vi "Parse Core.vi"(0 "SG Path in":refnum<class "SG 18GHz Path.lvclass">, 5 "Config Row":string[](array[string]), 11 "error in":errorcluster) -> (4 "SG Path out":refnum<class "SG 18GHz Path.lvclass">, 15 "error out":errorcluster)   [LabVIEW 2023, in "RFFixtureCharact.RFPM.lvlib" / "SG 18GHz Path.lvclass"]
uses:
  SG 18GHz Path.lvclass
  C:/srd-semi-rfcal-software/AuxTools/STSRFFixtureCharactUtility/Source/Code Modules/Common/Base Classes/Path/Path.lvclass
  Charact Result Accessor/Scalar/Scalar Charact Result Accessor.lvclass
  C:/srd-semi-rfcal-software/AuxTools/STSRFFixtureCharactUtility/Source/Code Modules/Fixture/RFPM/Charact Result Accessor/Base/Charact Result Accessor.lvclass
  C:/srd-semi-rfcal-software/AuxTools/STSRFFixtureCharactUtility/Source/Code Modules/Common/Result Accessor/Result Accessor.lvclass
  Common/Base Classes/Path/Path.lvclass/Path.ctl
  Common/Base Classes/Path/Properties/Read Date.vi
  Common/Base Classes/Path/Properties/Read Interval.vi
  Common/Data Cache/Settings Dictionary/Setting Keys.vi
  Public/Base Classes/Scalar/SG Abstract Path/SG Abstract Path.lvclass
  Common/RFCalAndFixtureCharact.Common.lvlib
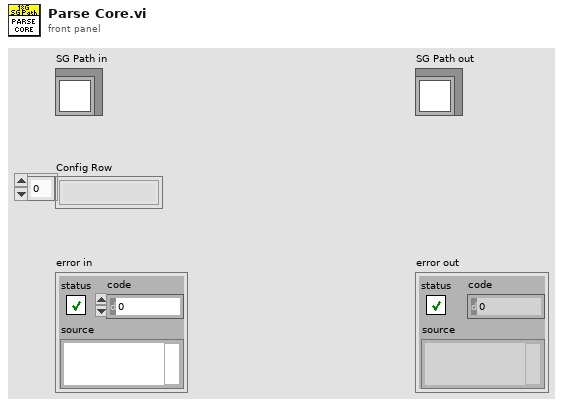
[diagram p1: front panel]
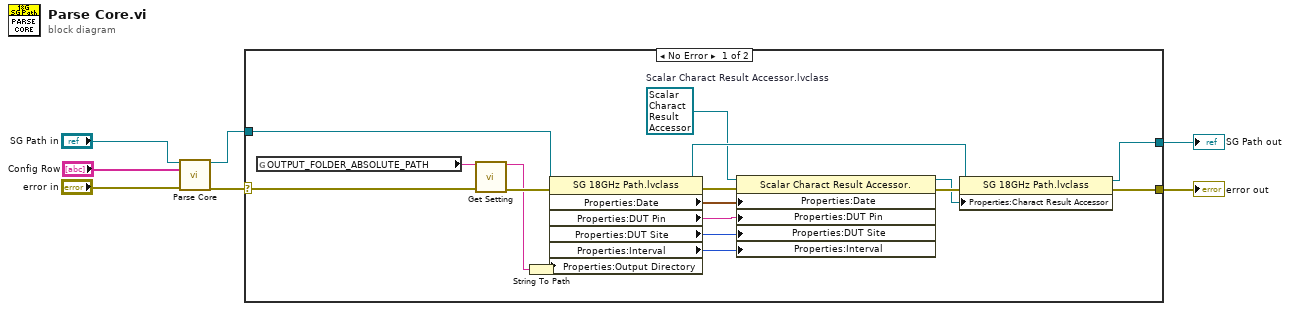
[diagram p0: block diagram]
diagram:
  n1 = call-parent "Parse Core.vi"("Scalar Path in"="SG Path in", "Config Row"="Config Row", "error in (no error)"="error in") -> ("Scalar Path out"=w3:refnum<class "SG 18GHz Path.lvclass">, "error out"=w4:errorcluster)  [unwired: 11 in]
  n2 = case shown="No Error" w4 {
    selector: w4 -> [w12 w25]
    tunnel: w3 -> [w14 w26]
    tunnel: [w15 w25] -> w2
    tunnel: [w13 w26] -> w1
    frame No Error {
      w16 = refnum<class "Scalar Charact Result Accessor.lvclass"> refnum  # Scalar Charact Result Accessor.lvclass
      n3 = global read "Setting Keys.vi" "OUTPUT_FOLDER_ABSOLUTE_PATH"() -> (w10:string)
      n4 = call "Get Setting.vi"("Setting name"=w10, "error in (no error)"=w12) -> ("Setting value out"=w8:string, "error out"=w11:errorcluster)  [unwired: 11 in, 1 out]
      n5 = String To Path(string=w8) -> (path=w9:path)
      n6 = property class="SG 18GHz Path.lvclass"(reference=w14, error in=w11, "Properties:Output Directory"=w9) -> (reference out=w18:refnum<class "SG 18GHz Path.lvclass">, error out=w23:errorcluster, "Properties:Date"=w22:timestamp, "Properties:DUT Pin"=w21:string, "Properties:DUT Site"=w20:i32, "Properties:Interval"=w19:i32)
      n7 = property class="Scalar Charact Result Accessor."(reference=w16, error in=w23, "Properties:Date"=w22, "Properties:DUT Pin"=w21, "Properties:DUT Site"=w20, "Properties:Interval"=w19) -> (reference out=w17:refnum<class "Scalar Charact Result Accessor.lvclass">, error out=w24:errorcluster)
      n8 = property class="SG 18GHz Path.lvclass"(reference=w18, error in=w24, "Properties:Charact Result Accessor"=w17) -> (reference out=w13:refnum<class "SG 18GHz Path.lvclass">, error out=w15:errorcluster)
    }
    frame Error {
    }
  }
  "error out" <- w2
  "SG Path out" <- w1
